vi "fgv_overlayrefs.vi"(7 "cmd":enum16{"read", "write"}(ring), 11 "overlayrefs":refnum<k24>[](array[refnum])) -> (3 "overlayrefs out":refnum<k24>[](array[refnum]))   [LabVIEW 2019]
uses:
  dll/GMap.NET.WindowsForms.dll
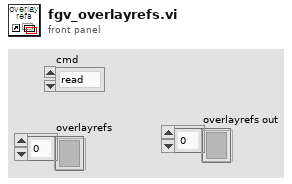
[diagram p1: front panel]
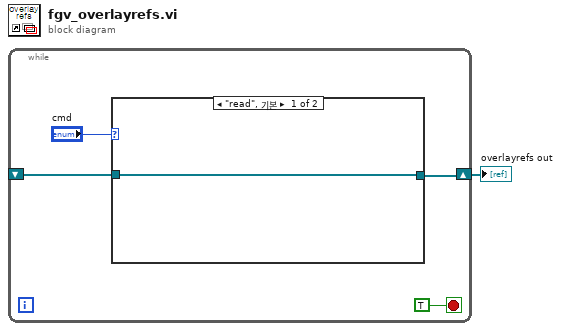
[diagram p0: block diagram]
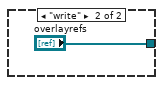
[diagram p2: hidden frame]
diagram:
  n1 = while {
    shift-right: [w3] -> w1
    shift-left: _ -> [w2]
    stop <- TRUE stop-if-true
    n2 = case shown="\"read\", 기본" "cmd" {
      tunnel: [w6 "overlayrefs"] -> w3
      tunnel: w2 -> [w6 _]
      frame "read", Default {
      }
      frame "write" {
      }
    }
  }
  "overlayrefs out" <- w1
